vi "BinArrayCreation.vi"(8 "error in (no error)":errorcluster, 11 "Histogram Bins":string[][](table)=[["0", "10"], ["10", "20"], ["20", "30"], ["30", "40"]]) -> (0 "error out":errorcluster, 2 "Lower Bounds":dbl[](array[numeric]), 3 "Upper Bounds":dbl[](array[numeric]))   [LabVIEW 2012, in "Histogram Custom Device.lvlib"]
uses:
  Histogram Custom Device.lvlib
panel:
  out "Problem with bins":bool
  in  "Done?":bool
  # "Lower Limits"
  # "Upper Limits"
  # "*Bins must stretch over a \ncontinuous numeric range"
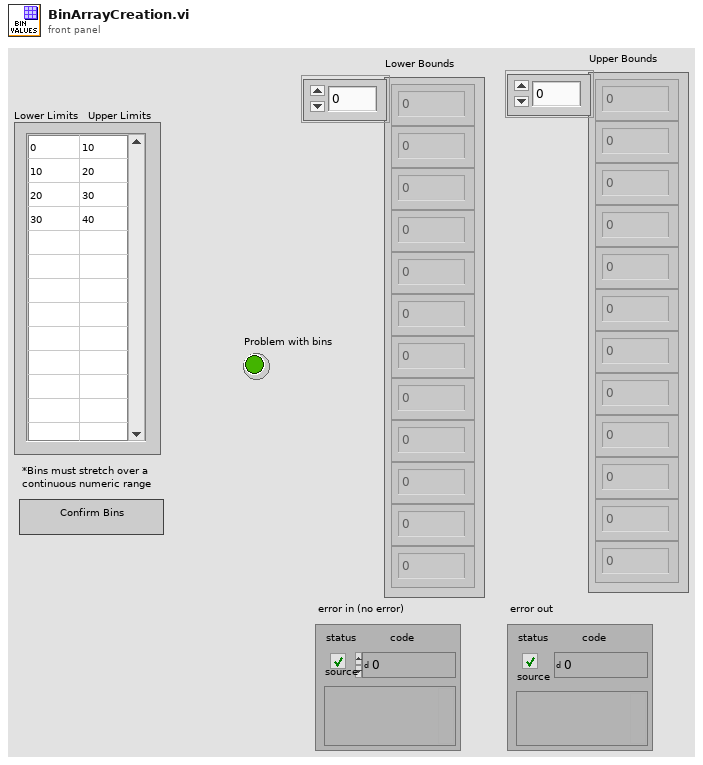
[diagram p1: front panel]
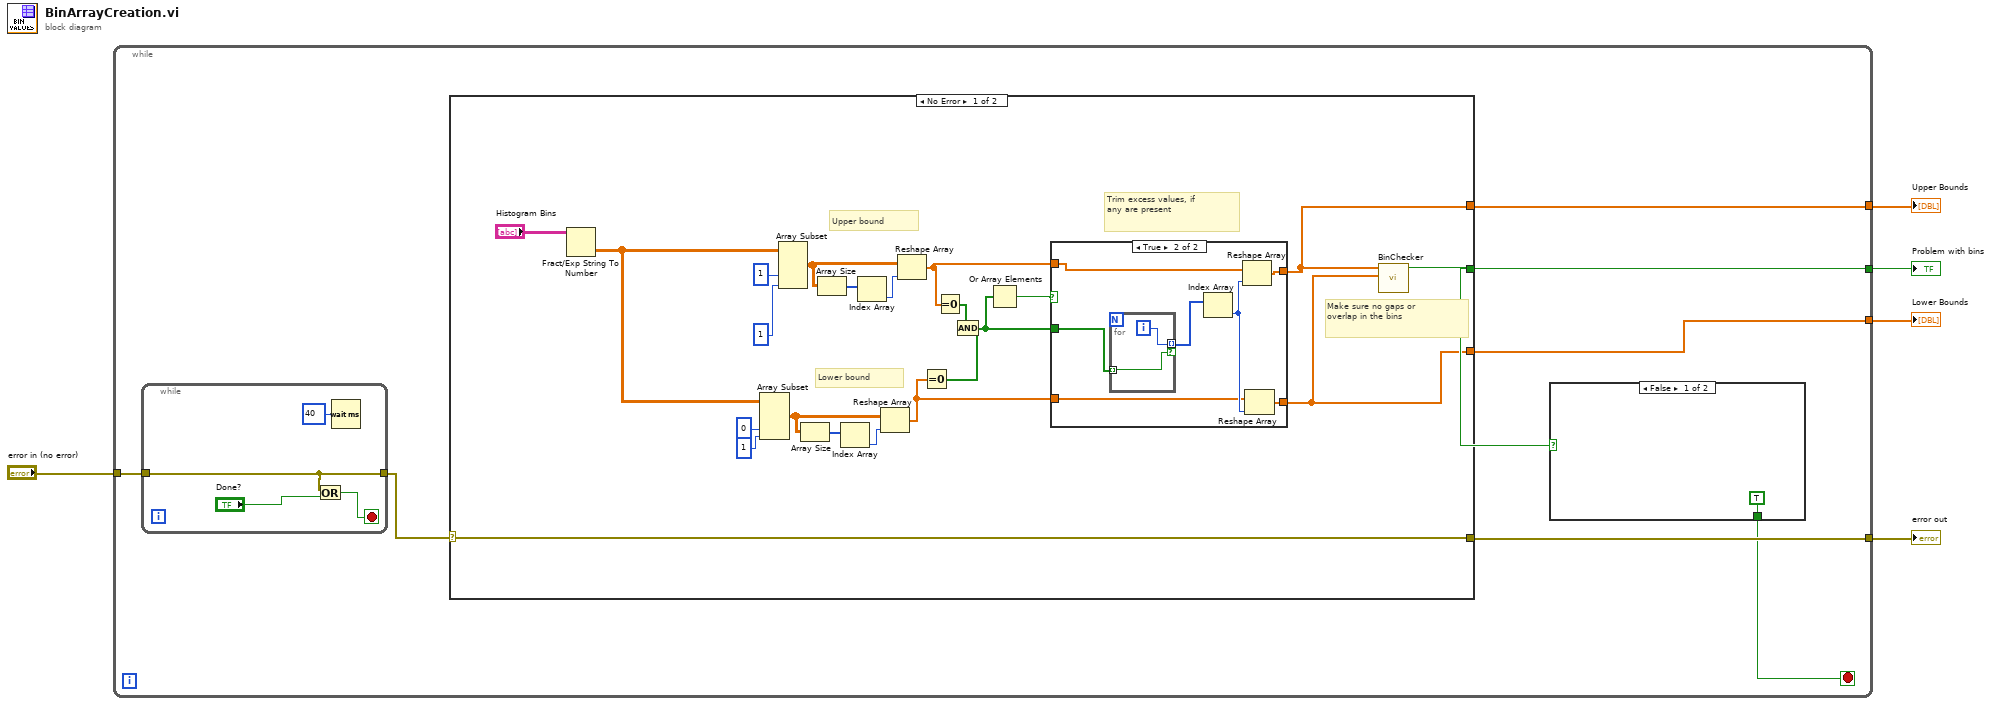
[diagram p0: block diagram]
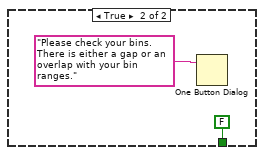
[diagram p2: hidden frame]
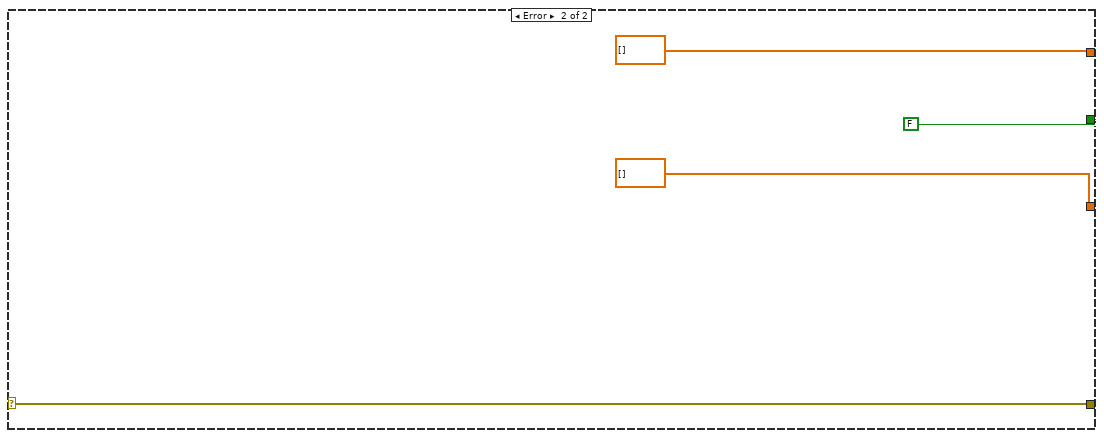
[diagram p4: hidden frame]
diagram:
  n1 = while {
    tunnel: [w12] -> w5
    tunnel: [w11] -> w1
    tunnel: [w10] -> w2
    tunnel: [w7] -> w4
    tunnel: "error in (no error)" -> [w8]
    stop <- w6 stop-if-true
    n2 = while {
      tunnel: w8 -> [w19]
      tunnel: [w19] -> w9
      stop <- w17 stop-if-true
      n3 = Or(x=w19, y="Done?") -> (x .or. y?=w17:bool)
      n4 = Wait (ms)(milliseconds to wait=u32 40) -> ()  [unwired: 1 out]
    }
    n5 = case shown="No Error" w9 {
      selector: w9 -> [w41 w56]
      tunnel: [w41 w56] -> w12
      tunnel: [w30 dbl[] []] -> w10
      tunnel: [w22 dbl[] []] -> w11
      tunnel: [w40 FALSE] -> w7
      frame No Error {
        # "Trim excess values, if\nany are present"
        # "Upper bound"
        # "Lower bound"
        # "Make sure no gaps or \noverlap in the bins"
        n6 = Fract/Exp String To Number(string="Histogram Bins") -> (number=w28:dbl[][])  [unwired: 3 in, 1 out]
        n7 = Array Subset(array=w28, index (col)=0 ("index"), length (col)=1 ("length")) -> (w33:dbl[][])  [unwired: 2 in]
        n8 = Array Subset(array=w28, index (col)=1 ("index"), length (col)=1 ("length")) -> (w34:dbl[][])  [unwired: 2 in]
        n9 = Array Size(array=w33) -> (size(s)=w25:i32[])
        n10 = Array Size(array=w34) -> (size(s)=w27:i32[])
        n11 = Index Array(array=w25) -> (element=w24:i32)  [unwired: 1 in]
        n12 = Index Array(array=w27) -> (element=w26:i32)  [unwired: 1 in]
        n13 = Reshape Array(w33, w24) -> (w23:dbl[])
        n14 = Reshape Array(w34, w26) -> (w39:dbl[])
        n15 = Equal To 0?(x=w23) -> (x = 0?=w38:bool[])
        n16 = Equal To 0?(x=w39) -> (x = 0?=w37:bool[])
        n17 = And(x=w37, y=w38) -> (x .and. y?=w21:bool[])
        n18 = Or Array Elements(Boolean array=w21) -> (logical OR=w20:bool)
        n19 = case shown="True" w20 {
          tunnel: w39 -> [w43 w48]
          tunnel: [w43 w47] -> w30
          tunnel: w23 -> [w42 w46]
          tunnel: [w42 w45] -> w22
          tunnel: w21 -> [_ w44]
          frame False {
          }
          frame True {
            n20 = for {
              tunnel: w44 -> [w51] mode=indexing
              tunnel: [w52] -> w49 mode=indexing if=w51
              i -> [w52]
            }
            n21 = Index Array(array=w49) -> (element=w50:i32)  [unwired: 1 in]
            n22 = Reshape Array(w48, w50) -> (w47:dbl[])
            n23 = Reshape Array(w46, w50) -> (w45:dbl[])
          }
        }
        n24 = call "BinChecker.vi"("Lower Bins"=w22, "Upper Bins"=w30) -> ("Boolean"=w40:bool)  [unwired: 9 in]
      }
      frame Error {
      }
    }
    n25 = case shown="False" w7 {
      tunnel: [TRUE FALSE] -> w6
      frame False {
      }
      frame True {
        n26 = One Button Dialog(message="Please check your bins. There is either a gap or an overlap with your bin ranges.") -> ()  [unwired: 1 in, 1 out]
      }
    }
  }
  "error out" <- w5
  "Problem with bins" <- w4
  "Upper Bounds" <- w2
  "Lower Bounds" <- w1
